vi "FRCts20_WebMethods_Convert_Requests.vi"(8 "error in (no error)":errorcluster, 11 "Request":T3) -> (0 "error out":errorcluster, 3 "output cluster":T1)   [LabVIEW 2014, in "FRCts20_WebMethods.lvlib"]
uses:
  FRCts20_WebMethods.lvlib
  Web Method Public Interface/FRCts20_WebMethods_ctl_request.ctl
  Backend/source/VI Source/FRCts20_Backend_API/FRCts20_Backend_API_Status.ctl
  Backend/source/VI Source/FRCts20_Backend_API/FRCts20_Backend_API_RequestRoot.ctl
  Backend/source/VI Source/FRCts20_Backend_API/FRCts20_Backend_API.lvlib
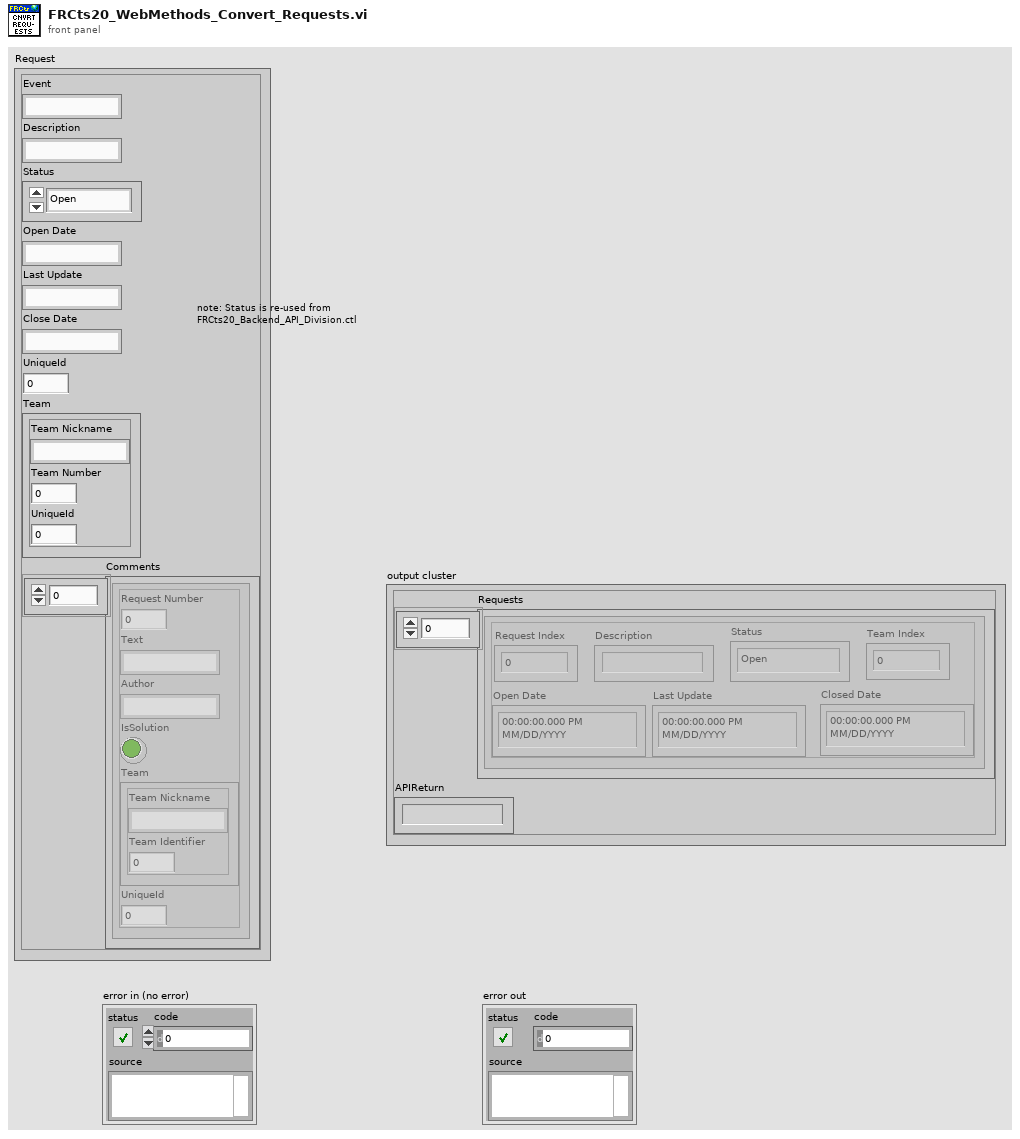
[diagram p1: front panel]
types:
  T1 = typedef "FRCts20_Backend_API.lvlib/FRCts20_Backend_API_RequestRoot.ctl" = cluster{"Requests":cluster{"Request Index":u32, "Description":string, "Status":T2, "Open Date":timestamp, "Last Update":timestamp, "Closed Date":timestamp, "Team Index":u32}[], "APIReturn":string}
  T2 = typedef "FRCts20_Backend_API.lvlib/FRCts20_Backend_API_Status.ctl" = enum16{"Open", "In Work", "Closed"}
  T3 = typedef "FRCts20_WebMethods.lvlib/FRCts20_WebMethods_ctl_request.ctl" = cluster{"Event":string, "Description":string, "Status":T2, "Open Date":string, "Last Update":string, "Close Date":string, "UniqueId":i32, "Team":cluster{"Team Nickname":string, "Team Number ":i32, "UniqueId":i32}, "Comments":cluster{"Request Number":dbl, "Text":string, "Author":string, "IsSolution":bool, "Team":cluster{"Team Nickname":string, "Team Identifier ":dbl}, "UniqueId":i32}[]}
  T4 = cluster{"Request Index":u32, "Description":string, "Status":T2, "Open Date":timestamp, "Last Update":timestamp, "Closed Date":timestamp, "Team Index":u32}[]
  T5 = cluster{"Request Index":u32, "Description":string, "Status":T2, "Open Date":timestamp, "Last Update":timestamp, "Closed Date":timestamp, "Team Index":u32}
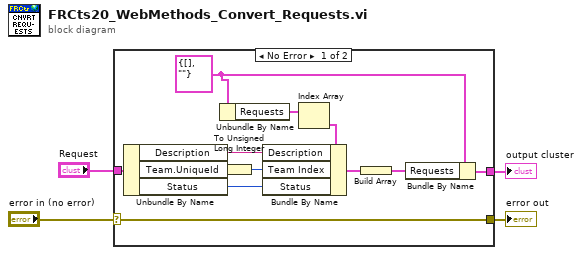
[diagram p0: block diagram]
diagram:
  n1 = case shown="No Error" "error in (no error)" {
    selector: "error in (no error)" -> [w16 w17]
    tunnel: [w8 _] -> w1
    tunnel: "Request" -> [w15 _]
    tunnel: [w16 w17] -> w4
    frame No Error {
      w7 = T1 {"Requests"=[], "APIReturn"=""} ("Request In")
      n2 = Unbundle By Name(w15) -> ("Description"=w14:string, "Team.UniqueId"=w12:i32, "Status"=w13:T2)
      n3 = Unbundle By Name(w7) -> ("Requests"=w6:T4)
      n4 = To Unsigned Long Integer(number=w12) -> (unsigned 32bit integer=w11:u32)
      n5 = Index Array(array=w6) -> (element=w5:T5)  [unwired: 1 in]
      n6 = Bundle By Name(cluster=w5, "Description"=w14, "Team Index"=w11, "Status"=w13) -> (w10:T5)
      n7 = Build Array(w10) -> (w9:T4)
      n8 = Bundle By Name(cluster=w7, "Requests"=w9) -> (w8:T1)
    }
    frame Error {
    }
  }
  "error out" <- w4
  "output cluster" <- w1
